vi "float64Array.vi"(3 "Array Length":i32=-1, 4 "Array":dbl[](array[numeric]), 5 "msg in":string) -> (2 "msg out":string)   [LabVIEW 2014]
doc: "Flattens an float64 array into a message"
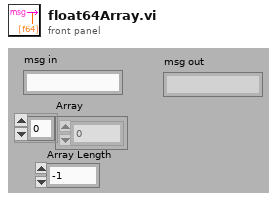
[diagram p1: front panel]
types:
  T1 = enum16{"big-endian, network order", "native, host order", "little-endian"}
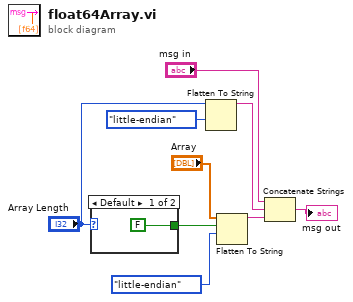
[diagram p0: block diagram]
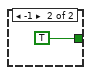
[diagram p2: hidden frame]
diagram:
  n1 = case shown="Default" "Array Length" {
    tunnel: [FALSE TRUE] -> w5
    frame Default {
    }
    frame -1 {
    }
  }
  n2 = Flatten To String(anything="Array Length", byte order (0:big-endian, network order)=T1."little-endian") -> (data string=w1:string)  [unwired: 2 in, 2 out]
  n3 = Flatten To String(anything="Array", prepend array or string size? (T)=w5, byte order (0:big-endian, network order)=T1."little-endian") -> (data string=w8:string)  [unwired: 1 in, 2 out]
  n4 = Concatenate Strings("msg in", w1, w8) -> (→"msg out":string)
